vi "Input Channels by Type.vi"(11 "Voicemeeter Type":T1) -> (2 "Channel Count":i32[](array[numeric]))   [LabVIEW 2022 SP3, in "VoiceMeeterRemote.lvlib"]
uses:
  VoiceMeeterRemote.lvlib
  Voicemeeter Type.ctl
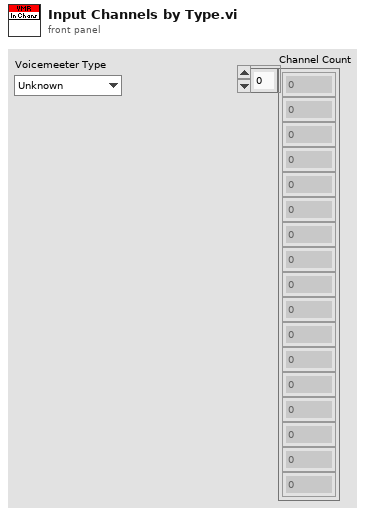
[diagram p1: front panel]
types:
  T1 = typedef "VoiceMeeterRemote.lvlib/Voicemeeter Type.ctl" = enum16{"Unknown", "Voicemeeter", "Banana", "Potato", "Potato x64"}
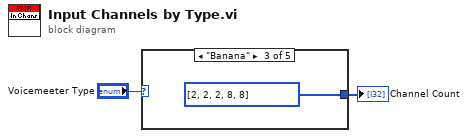
[diagram p0: block diagram]
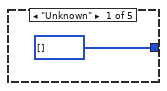
[diagram p2: hidden frame]
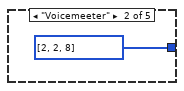
[diagram p3: hidden frame]
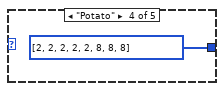
[diagram p4: hidden frame]
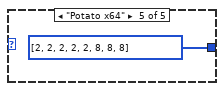
[diagram p5: hidden frame]
diagram:
  n1 = case shown="\"Banana\"" "Voicemeeter Type" {
    tunnel: [i32[] [] i32[] [2, 2, 8] i32[] [2, 2, 2, 8, 8] i32[] [2, 2, 2, 2, 2, 8, 8, 8] i32[] [2, 2, 2, 2, 2, 8, 8, 8]] -> w1
    frame "Unknown" {
    }
    frame "Voicemeeter" {
    }
    frame "Banana" {
    }
    frame "Potato" {
    }
    frame "Potato x64" {
    }
  }
  "Channel Count" <- w1
